vi "Write Current Command Code.vi"(8 "error in (no error)":errorcluster, 10 "Current Command Code":string, 11 "AK RS232 in":refnum<class "AK RS-xxx.lvclass">) -> (0 "error out":errorcluster, 3 "AK RS232 out":refnum<class "AK RS-xxx.lvclass">)   [LabVIEW 2013, in "Protocol Classes.lvlib" / "AK RS-xxx.lvclass"]
uses:
  AK RS-xxx.lvclass
  AK RS-xxx.lvclass/AK RS-xxx.ctl
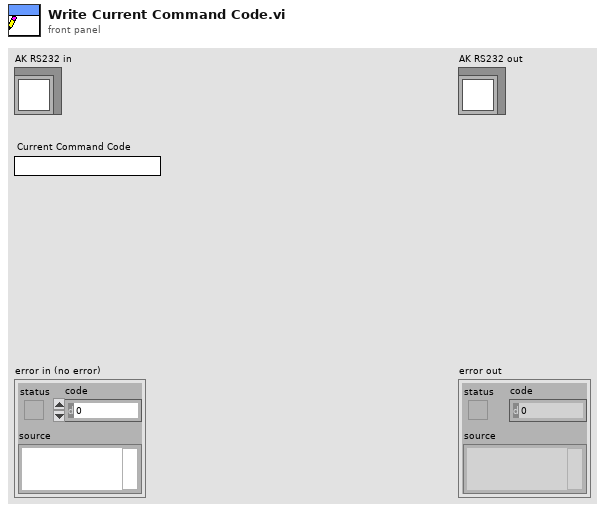
[diagram p1: front panel]
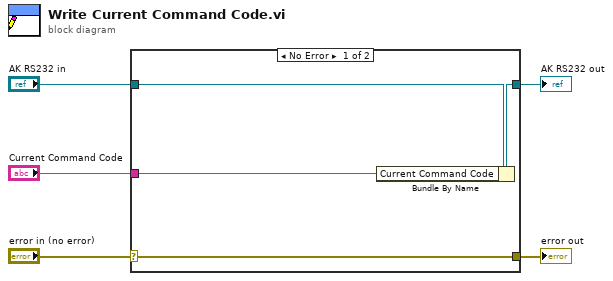
[diagram p0: block diagram]
diagram:
  n1 = case shown="No Error" "error in (no error)" {
    selector: "error in (no error)" -> [w9 w10]
    tunnel: [w9 w10] -> w4
    tunnel: [w7 w11] -> w2
    tunnel: "AK RS232 in" -> [w8 w11]
    tunnel: "Current Command Code" -> [w6 _]
    frame No Error {
      n2 = Bundle By Name(cluster=w8, "Current Command Code"=w6) -> (w7:refnum<class "AK RS-xxx.lvclass">)
    }
    frame Error {
    }
  }
  "error out" <- w4
  "AK RS232 out" <- w2
